vi "LS218_Init.vi"(0 "VISA":refnum<visa-resource-name>, 7 "Reset (T: Reset)":bool, 9 "Reset Defaults (F:Dont Reset)":bool, 11 "error in (no error)":errorcluster, 12 "call-VISA-Close":T1=enum."CALL CLOSE") -> (4 "VISA Out":refnum<visa-resource-name>="COM1", 6 "Reply":string="\nLSCI,MODEL218E,221094,042109\r", 15 "error out":errorcluster)   [LabVIEW 2012, in "Lake Shore Cryotronics 218.lvlib"]
doc: "modified for HARPSN\n\nThis VI passes the addressing information in the instrument decriptor to the Instr Open VI and returns the instrument ID. You can optionally reset the instrument by setting the front panel reset control. You must run this VI before using any of the instrument driver VIs for this instrument.\n\nNOTE: If you do not want the instrument reset to its default setup state you MUST set the Reset Defaults control to FALSE."
uses:
  <instrlib>/Lake Shore Cryotronics 218/Lake Shore Cryotronics 218.lvlib
  Common/Call-VISA-Close.ctl
panel:
  # "Check\nDon't Check"
  # "Reset\nDon't Reset"
  # "Reset to Default State\nDon't Reset to Default State"
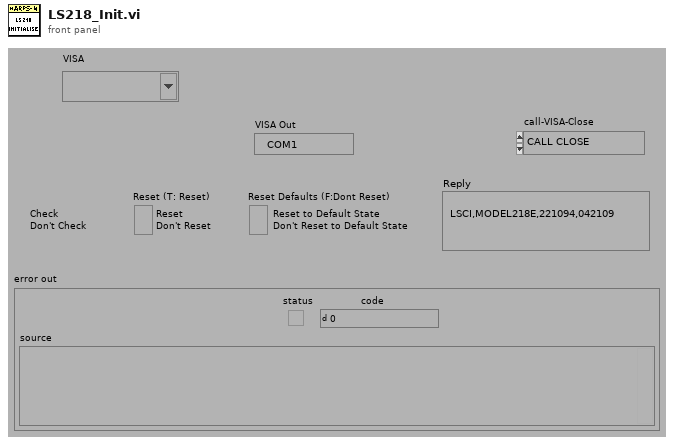
[diagram p1: front panel]
types:
  T1 = typedef "Call-VISA-Close.ctl" = enum16{"DON'T CALL", "CALL CLOSE"}
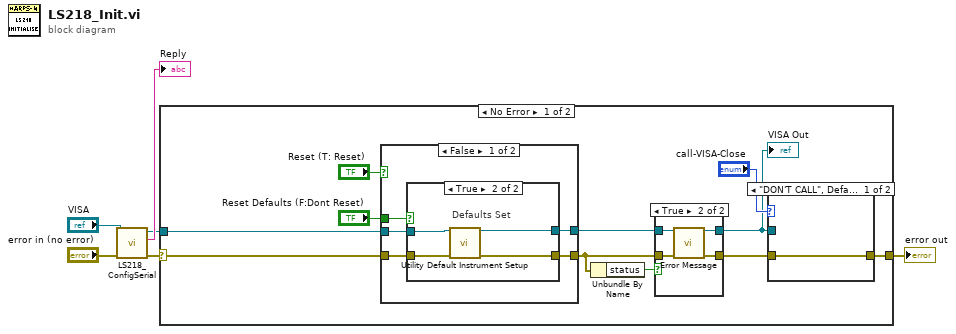
[diagram p0: block diagram]
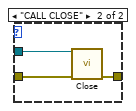
[diagram p2: hidden frame]
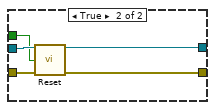
[diagram p5: hidden frame]
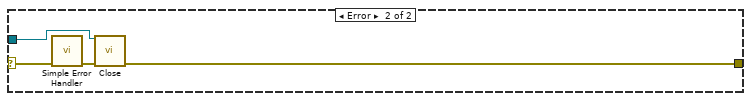
[diagram p6: hidden frame]
diagram:
  n1 = call "LS218_ConfigSerial.vi"("error in"="error in (no error)", "VISA"="VISA") -> ("error out"=w2:errorcluster, "ID String"=→"Reply":string, "VISA Out"=w3:refnum<visa-resource-name>)  [unwired: 4 in]
  n2 = case shown="No Error" w2 {
    selector: w2 -> [w7 w47]
    tunnel: w3 -> [w17 w46]
    tunnel: [w9 w44] -> w6
    frame No Error {
      n3 = case shown="False" "Reset (T: Reset)" {
        tunnel: w7 -> [w31 w40]
        tunnel: [w30 w43] -> w15
        tunnel: w17 -> [w32 w41]
        tunnel: [w29 w42] -> w14
        tunnel: "Reset Defaults (F:Dont Reset)" -> [w28 w39]
        frame False {
          n4 = case shown="True" w28 {
            tunnel: w32 -> [w34 w38]
            tunnel: w31 -> [w33 w37]
            tunnel: [w33 w36] -> w30
            tunnel: [w34 w35] -> w29
            frame False {
              # "No Defaults Set"
            }
            frame True {
              # "Defaults Set"
              n5 = call <instrlib>:"Utility Default Instrument Setup.vi"("VISA resource name"=w38, "error in (no error)"=w37) -> ("VISA resource name out"=w35:refnum<visa-resource-name>, "error out"=w36:errorcluster)  [unwired: 12 in]
            }
          }
        }
        frame True {
          n6 = call <instrlib>:"Reset.vi"("VISA resource name"=w41, "Reset Defaults (F:Dont Reset)"=w39, "error in (no error)"=w40) -> ("VISA resource name out"=w42:refnum<visa-resource-name>, "error out"=w43:errorcluster)  [unwired: 11 in]
        }
      }
      n7 = Unbundle By Name(w15) -> ("status"=w16:bool)
      n8 = case shown="True" w16 {
        tunnel: w14 -> [w23 w27]
        tunnel: w15 -> [w22 w26]
        tunnel: [w23 w25] -> w10
        tunnel: [w22 w24] -> w11
        frame False {
        }
        frame True {
          n9 = call <instrlib>:"Error Message.vi"("VISA resource name"=w27, "error in (no error)"=w26) -> ("VISA resource name out"=w25:refnum<visa-resource-name>, "error out"=w24:errorcluster)  [unwired: 9 in, 3 out]
        }
      }
      "VISA Out" <- w10
      n10 = case shown="\"DON'T CALL\", Default" "call-VISA-Close" {
        tunnel: w11 -> [w18 w21]
        tunnel: w10 -> [_ w20]
        tunnel: [w18 w19] -> w9
        frame "DON'T CALL", Default {
        }
        frame "CALL CLOSE" {
          n11 = call <instrlib>:"Close.vi"("VISA resource name"=w20, "error in (no error)"=w21) -> ("error out"=w19:errorcluster)  [unwired: 13 in]
        }
      }
    }
    frame Error {
      n12 = call <vilib>:"Simple Error Handler.vi"("error in (no error)"=w47) -> ("error out"=w45:errorcluster)  [unwired: 4 in, 4 out]
      n13 = call <instrlib>:"Close.vi"("VISA resource name"=w46, "error in (no error)"=w45) -> ("error out"=w44:errorcluster)  [unwired: 13 in]
    }
  }
  "error out" <- w6
